vi "write_file_contents(SubVI).vi"(9 "레코드 3":T1(array[cluster]), 10 "레코드 입력":T1(array[cluster]), 11 "데이터로그 경로(대화 상자 사용)":path) -> ()   [LabVIEW 2018]
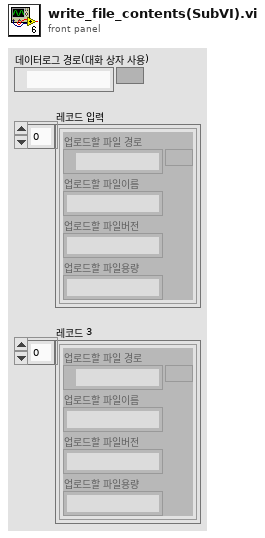
[diagram p1: front panel]
types:
  T1 = cluster{"업로드할 파일 경로":path, "업로드할 파일이름":string, "업로드할 파일버전":string, "업로드할 파일용량":string}[]
  T2 = enum16{"open", "replace", "create", "open or create", "replace or create", "replace or create with confirmation"}
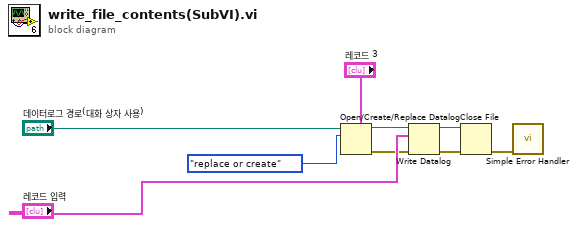
[diagram p0: block diagram]
diagram:
  n1 = Open/Create/Replace Datalog(5:"레코드 3", 10:T2."replace or create" ("동작(0:open)"), 11:"데이터로그 경로(대화 상자 사용)") -> (0:w5:errorcluster, 3:w1:refnum<k1>)  [unwired: 3 in, 1 out]
  n2 = Write Datalog(4:w5, 6:"레코드 입력", 7:w1) -> (0:w3:errorcluster, 3:w4:refnum<k1>)
  n3 = Close File(refnum=w4, error in=w3) -> (error out=w2:errorcluster)  [unwired: 1 out]
  n4 = call <vilib>:"Simple Error Handler.vi"("error in (no error)"=w2) -> ()  [unwired: 4 in, 5 out]
